vi "Condition Msg VI.vi"(8 "error in":errorcluster, 9 "Name Msg Strategy":string, 10 "Ref.Msg VI":refnum<vi>) -> (0 "error out":errorcluster)   [LabVIEW 2021, in "_Msg Rescript.lvlib" / "_Msg Rescript.lvclass"]
uses:
  _Msg Rescript.lvclass
  _Msg Rescript.lvclass/_Msg Rescript.ctl
  <vilib>/Utility/traverseref.llb/TRef TravTarget.ctl
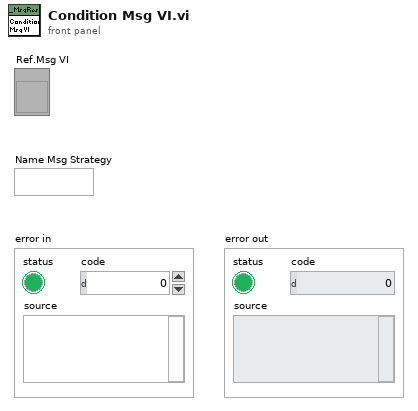
[diagram p1: front panel]
types:
  T1 = typedef "TRef TravTarget.ctl" = enum16{"FP", "BD", "Other"}
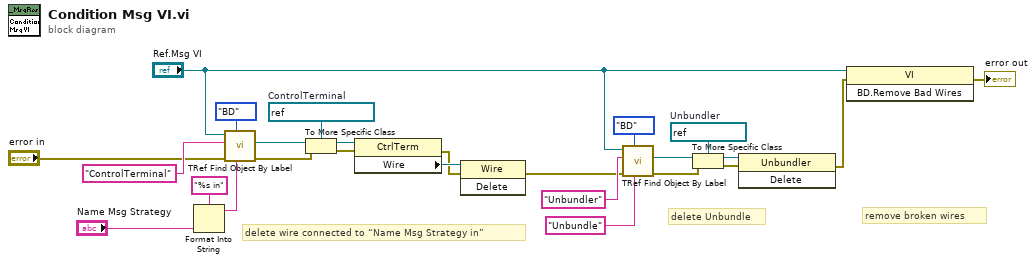
[diagram p0: block diagram]
diagram:
  w13 = refnum<vi> refnum  # Unbundler
  w21 = refnum<vi> refnum  # ControlTerminal
  # "remove broken wires"
  # "delete Unbundle"
  # "delete wire connected to “Name Msg Strategy in”"
  n1 = Format Into String(format string="%s in", "Name Msg Strategy") -> (resulting string=w20:string)  [unwired: 2 in, 1 out]
  n2 = call <vilib>:"TRef Find Object By Label.vi"("Label"=w20, "Traverse Target"=TRef_TravTarget."BD", "error in (no error)"="error in", "Class Name"="ControlTerminal", "VI Ref"="Ref.Msg VI") -> ("error out"=w24:errorcluster, "Found Obj Ref"=w25:refnum<vi>)  [unwired: 3 in, 2 out]
  n3 = To More Specific Class(target class=w21, reference=w25, error in=w24) -> (specific class reference=w18:refnum<vi>, error out=w17:errorcluster)
  n4 = property class="CtrlTerm"(reference=w18, error in=w17) -> (error out=w15:errorcluster, "Wire"=w16:refnum<vi>)  [unwired: 1 out]
  n5 = invoke class="Wire" method="Delete"(reference=w16, error in=w15) -> (error out=w8:errorcluster)  [unwired: 1 in, 2 out]
  n6 = call <vilib>:"TRef Find Object By Label.vi"("Label"="Unbundle", "Traverse Target"=TRef_TravTarget."BD", "error in (no error)"=w8, "Class Name"="Unbundler", "VI Ref"="Ref.Msg VI") -> ("error out"=w14:errorcluster, "Found Obj Ref"=w12:refnum<vi>)  [unwired: 3 in, 2 out]
  n7 = To More Specific Class(target class=w13, reference=w12, error in=w14) -> (specific class reference=w7:refnum<vi>, error out=w6:errorcluster)
  n8 = invoke class="Unbundler" method="Delete"(reference=w7, error in=w6) -> (error out=w5:errorcluster)  [unwired: 1 in, 2 out]
  n9 = invoke class="VI" method="BD.Remove Bad Wires"(reference="Ref.Msg VI", error in=w5) -> (error out=→"error out":errorcluster)  [unwired: 1 in, 2 out]
